vi "Example-I2C.vi"() -> ()   [LabVIEW 2018]
panel:
  in  "addr":u8=96 format="%.0x"
  out "数值":i32
  out "波形图":u8[](graph)
  out "SerialNumber":string
  out "rxcount out":i32
  out "rgRX":u8[](array[numeric])
  in  "Tx data":u8[](array[numeric])
  in  "SDA IO(0~15)":i32=1
  in  "SCL IO(0~15)":i32
  in  "Frequency(Hz)":i32(ring)=9600 items=["110"=110, "150"=150, "300"=300, "600"=600, "1200"=1200, "2400"=2400, "4800"=4800, "9600"=9600, "14400"=14400, "19200"=19200, "28800"=28800, "38400"=38400, "56000"=56000, "57600"=57600, "115200"=115200, "128000"=128000, "153600"=153600, "230400"=230400, "256000"=256000, "406800"=406800, "921600"=921600]
  out "returns":i32[](array[numeric])
  out "error out":errorcluster caption="错误输出"
  in  "error in (no error)":errorcluster caption="错误输入（无错误）"
  out "ftHandle out":u64=363562184
  in  "设备索引":i32
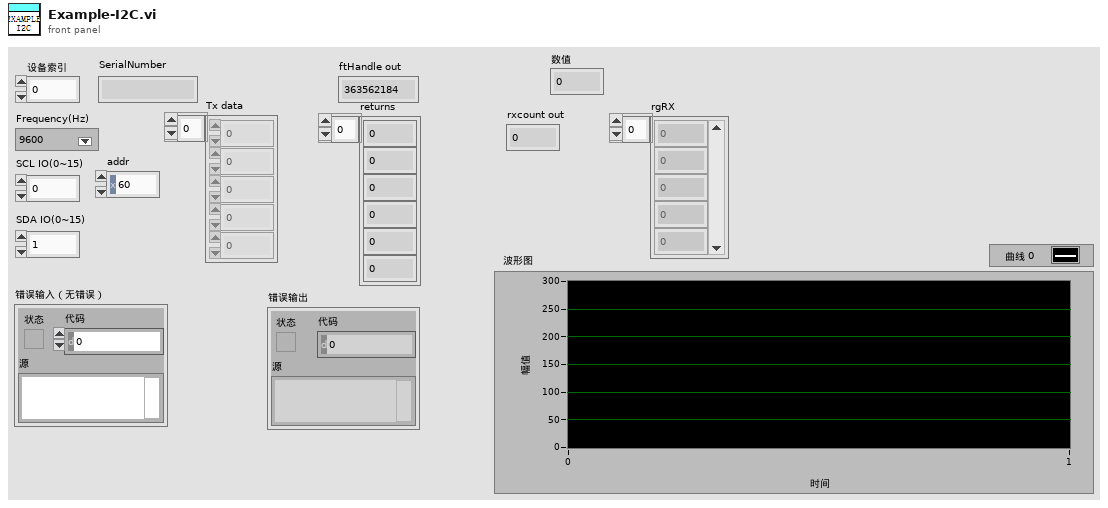
[diagram p1: front panel]
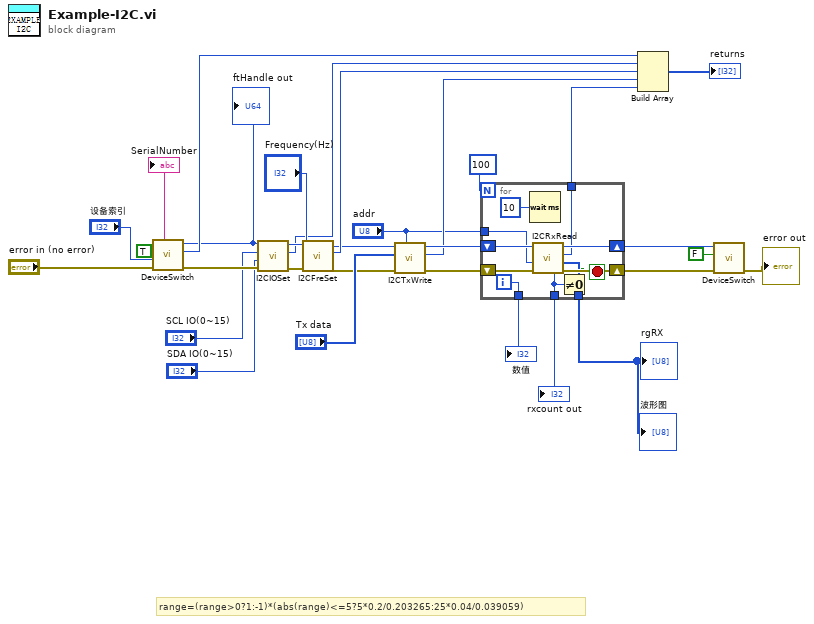
[diagram p0: block diagram]
diagram:
  # "range=(range>0?1:-1)*(abs(range)<=5?5*0.2/0.203265:25*0.04/0.039059)"
  n1 = call "DeviceSwitch.vi"("error in (no error)"="error in (no error)", "Device Index"="设备索引", "Open"=TRUE) -> ("error out"=w24:errorcluster, "function return"=w27:i32, "handle out"=w6:u64, "SerialNumber"=→"SerialNumber":string)  [unwired: 4 in, 1 out]
  "ftHandle out" <- w6
  n2 = call "I2CIOSet.vi"("error in (no error)"=w24, "SDA IO(0~15)"="SDA IO(0~15)", "SCL IO(0~15)"="SCL IO(0~15)", "handle"=w6) -> ("error out"=w23:errorcluster, "function return"=w18:i32, "handle out"=w19:u64)  [unwired: 5 in]
  n3 = call "I2CFreSet.vi"("error in (no error)"=w23, "Frequency(Hz)"="Frequency(Hz)", "handle"=w19) -> ("error out"=w13:errorcluster, "function return"=w17:i32, "handle out"=w16:u64)  [unwired: 6 in]
  n4 = call "I2CTxWrite.vi"("addr"="addr", "error in (no error)"=w13, "data"="Tx data", "handle"=w16) -> ("error out"=w14:errorcluster, "function return"=w9:i32, "handle out"=w10:u64)  [unwired: 5 in]
  n5 = for {
    N: 100 -> [_]
    tunnel: [w38] -> w8
    tunnel: [w37] -> w3
    tunnel: [w36] -> w5
    shift-right: [w41] -> w12
    shift-left: w14 -> [w42]
    shift-right: [w40] -> w11
    shift-left: w10 -> [w39]
    tunnel: [w33] -> w2
    tunnel: "addr" -> [w32]
    i -> [w33]
    stop <- w35 stop-if-true
    n6 = Wait (ms)(milliseconds to wait=u32 10 ("等待时间（毫秒）")) -> ()  [unwired: 1 out]
    n7 = call "I2CRxRead.vi"("error in (no error)"=w42, "addr"=w32, "handle"=w39) -> ("error out"=w41:errorcluster, "rgRX"=w37:u8[], "function return"=w38:i32, "handle out"=w40:u64, "rxcount out"=w36:i32)  [unwired: 4 in]
    n8 = Not Equal To 0?(x=w36) -> (x != 0?=w35:bool)
  }
  "rgRX" <- w3
  "rxcount out" <- w5
  "波形图" <- w3
  "数值" <- w2
  n9 = Build Array(w27, w18, w17, w9, w8) -> (→"returns":i32[])
  n10 = call "DeviceSwitch.vi"("error in (no error)"=w12, "Open"=FALSE, "handle"=w11) -> ("error out"=→"error out":errorcluster)  [unwired: 4 in, 4 out]
